vi "verifyLegalMoves.vi"(8 "error in (no error)":errorcluster, 10 "Index":variant, 11 "object in":refnum<class "Board.lvclass">) -> (0 "error out":errorcluster, 3 "object out":refnum<class "Board.lvclass">)   [LabVIEW 2020, in "Board.lvclass"]
uses:
  Board.lvclass
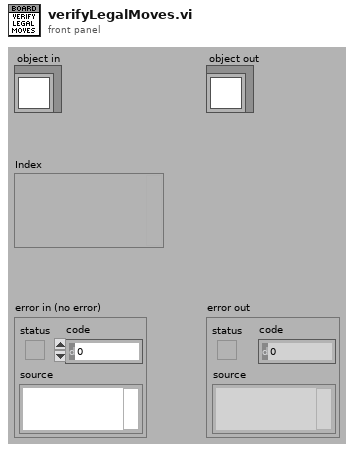
[diagram p1: front panel]
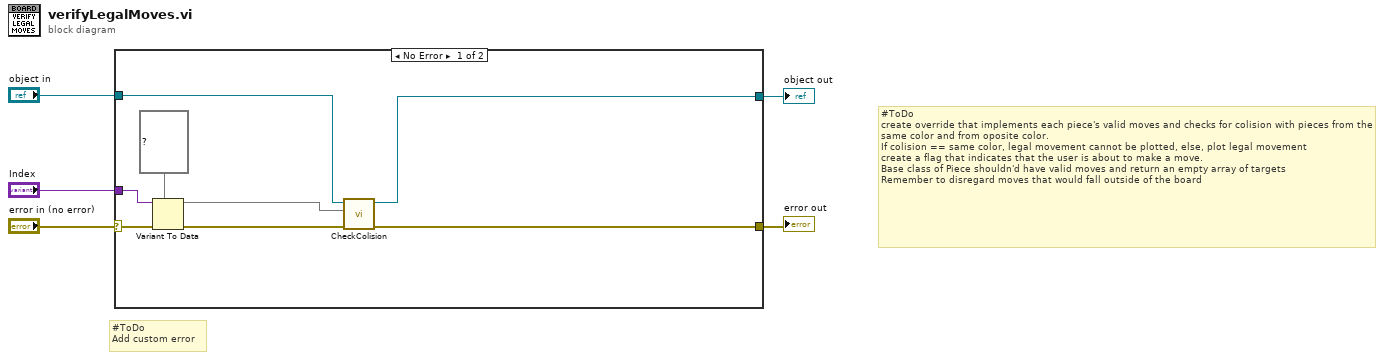
[diagram p0: block diagram]
diagram:
  # "#ToDo\nAdd custom error"
  # "#ToDo\ncreate override that implements each piece's valid moves and checks for colision with pieces from the same color and from oposite color.\nIf colision == same color, legal movement cannot be plotted, else, plot legal movement\ncreate a flag that indicates that the user is about to make a move.\nBase class of Piece shouldn'd have valid moves and return an empty array of targets\nRemember to disregard moves that would fall outside of the board"
  n1 = case shown="No Error" "error in (no error)" {
    selector: "error in (no error)" -> [w13 w15]
    tunnel: [w8 w15] -> w4
    tunnel: [w7 w14] -> w2
    tunnel: "object in" -> [w10 w14]
    tunnel: "Index" -> [w12 _]
    frame No Error {
      n2 = Variant To Data(error in=w13, type=map{string, i32} {} ("key"), Variant=w12) -> (data=w6:map{string, i32}, error out=w11:errorcluster)
      n3 = call "CheckColision.vi"("error in (no error)"=w11, "Clicked Square"=w6, "object in"=w10) -> ("error out"=w8:errorcluster, "object out"=w7:refnum<class "Board.lvclass">)  [unwired: 7 in]
    }
    frame Error {
    }
  }
  "error out" <- w4
  "object out" <- w2
